vi "PH_PPMA_PowerUnit.src Rods.vi"(0 "i ref in":refnum<vi>, 5 "error in (no error)":errorcluster) -> (14 "i ref out":refnum<vi>, 19 "error out":errorcluster)   [LabVIEW 2014, in "PH_PPMA_PowerUnit.lvlib"]
doc: "This is the action VI of the _StateDumpRoss event case. It checks the \"State Rel Rods\". If this is\n\n1 (rel Rods up): if State SM = Close Dump Rods and Remote Controlled by = N/A, an state change request is send to SM to get \"Wait on Shot Cmd\"\n\n2 (rel Rods down): if State SM = Open Dump Rods and Remote Controlled by = N/A and State RR = on (open) and Iginitron.State Device = on and State PSU = off, an state change request is send to SM to get \"Close Ross Relais\". \n\nFinally it allways calls \"State PU\"."
uses:
  PH_PPMA_PowerUnit.lvlib
  PH_Basics/PH_PowerUnit_BaseClass/PH_PowerUnit_BaseClass.SM States.ctl
  PH_Basics/PH_StatusHandler/PH_StatusHandler.Status.ctl
  PH_Basics/PH_PowerUnit_BaseClass/PH_PowerUnit_BaseClass.lvlib
  PH_Basics/PH_StatusHandler/PH_StatusHandler.lvlib
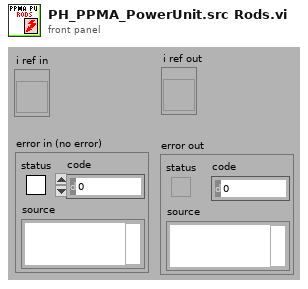
[diagram p1: front panel]
types:
  T1 = typedef "PH_PPMA_PowerUnit.lvlib/PH_PPMA_PowerUnit.i attribute.ctl" = cluster{"GUI Refs":cluster{"Rods":refnum<vi>, "Ignitron":refnum<vi>, "Rossrelais":refnum<vi>, "Set Voltage":refnum<vi>, "PSU":refnum<vi>, "EOC":refnum<vi>, "Trigger":refnum<vi>}, "Rods":T2, "PSU":T4, "Ross Relais":T5, "Ignitron":T6, "Trigger":cluster{"State Device":T3, "linked?":bool}, "Timing Settings":cluster{"Prdc Fast?":bool, "Default Value Periodic Interval":i32, "Mercury on since":dbl, "Warm up Time Mercury [s]":dbl}, "Set Voltage [V]":dbl}
  T2 = typedef "PH_PPMA_PowerUnit.lvlib/PH_PPMA_PowerUnit.Rods Attributes.ctl" = cluster{"Instancename":string, "Device Status":T3, "linked?":bool}
  T3 = typedef "PH_StatusHandler.lvlib/PH_StatusHandler.Status.ctl" = i16
  T4 = typedef "PH_PP_Common.lvlib/PH_PP_Common.PSU Attributes.ctl" = cluster{"lower limit [V]":dbl, "upper limit [V]":dbl, "Voltage set":bool, "State Device":T3, "linked?":bool}
  T5 = typedef "PH_PP_Common.lvlib/PH_PP_Common.Ross Relais Attributes.ctl" = cluster{"State Device":T3, "linked?":bool}
  T6 = typedef "PH_PP_Common.lvlib/PH_PP_Common.Ignitron Attributes.ctl" = cluster{"State Device":T3, "linked?":bool}
  T7 = typedef "PH_PowerUnit_BaseClass.lvlib/PH_PowerUnit_BaseClass.SM States.ctl" = enum16{".", "Stand by", "Switch PU on", "Configure", "Set Default Voltage", "Set STANDBY", "Set READY", "Wait for Shot Cmd", "Open Dump Rods", "Open Ross Relais", "Close Ross Relais", "Switch PSU on", "Switch PSU off", "Charge", "Switch GD Channel on", "Close Dump Rods", "Rods-TO", "RR-TO", "PSU-TO", "Trigger-TO"}
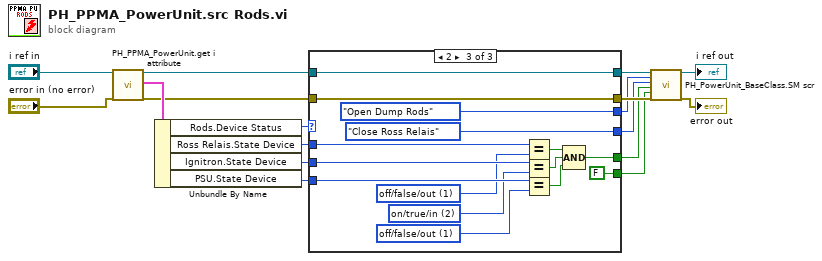
[diagram p0: block diagram]
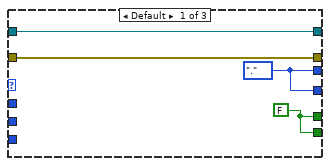
[diagram p2: hidden frame]
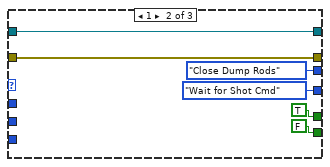
[diagram p3: hidden frame]
diagram:
  n1 = call "PH_PPMA_PowerUnit.get i attribute.vi"("i ref in"="i ref in", "error in (no error)"="error in (no error)") -> ("i ref out"=w14:refnum<vi>, "i attribute"=w17:T1, "error out"=w13:errorcluster)  [unwired: 15 in]
  n2 = Unbundle By Name(w17) -> ("Rods.Device Status"=w12:T3, "Ross Relais.State Device"=w11:T3, "Ignitron.State Device"=w10:T3, "PSU.State Device"=w9:T3)
  n3 = case shown="2" w12 {
    tunnel: w14 -> [w21 w23 w29]
    tunnel: w13 -> [w20 w22 w28]
    tunnel: [w20 w22 w28] -> w8
    tunnel: [w21 w23 w29] -> w6
    tunnel: w11 -> [_ _ w42]
    tunnel: w10 -> [_ _ w41]
    tunnel: w9 -> [_ _ w40]
    tunnel: [w19 PH_PowerUnit_BaseClass.SM_States."Close Dump Rods" ("Current SM State (condition)") PH_PowerUnit_BaseClass.SM_States."Open Dump Rods" ("Current SM State (condition)")] -> w4
    tunnel: [w19 PH_PowerUnit_BaseClass.SM_States."Wait for Shot Cmd" ("Current SM State (condition)") PH_PowerUnit_BaseClass.SM_States."Close Ross Relais" ("Current SM State (condition)")] -> w3
    tunnel: [w18 TRUE w31] -> w2
    tunnel: [w18 FALSE FALSE] -> w1
    frame Default {
      w18 = FALSE
      w19 = PH_PowerUnit_BaseClass.SM_States."." ("Current SM State (condition)")
    }
    frame 1 {
    }
    frame 2 {
      w34 = T3 1 items=["no info", "off/false/out", "on/true/in", "Failure", "Alarm", "Status 1", "Status 2", "Status 3"] ("PSU.State PSU")
      w35 = T3 2 items=["no info", "off/false/out", "on/true/in", "Failure", "Alarm", "Status 1", "Status 2", "Status 3"] ("Ignitron.State Device")
      w36 = T3 1 items=["no info", "off/false/out", "on/true/in", "Failure", "Alarm", "Status 1", "Status 2", "Status 3"] ("Ross Relais.State RR")
      n4 = Equal?(x=w42, y=w36) -> (x = y?=w39:bool)
      n5 = Equal?(x=w41, y=w35) -> (x = y?=w38:bool)
      n6 = Equal?(x=w40, y=w34) -> (x = y?=w37:bool)
      n7 = Compound Arithmetic op=AND(w39, w38, w37) -> (w31:bool)
    }
  }
  n8 = call "PH_PowerUnit_BaseClass.SM scr.vi"("VI in"=w6, "Current SM State (condition)"=w4, "Wanted SM State"=w3, "Further change condition"=w2, "PU in use is condition? (true)"=w1, "error in (no error)"=w8) -> ("VI out"=→"i ref out":refnum<vi>, "error out"=→"error out":errorcluster)  [unwired: 12 in]
